vi "sub vi - GET ALL TEMP v7.vi"(0 "LA01-EN":bool, 1 "LA02-EN":bool, 3 "LA03-EN":bool, 4 "LA04-EN":bool, 5 "LA05-EN":bool, 6 "simulate":bool, 7 "Gen Cal Value":dbl) -> (10 "LOOP TIME":dbl, 11 "Fault Counters":u64[](array[numeric]), 12 "ID":T1, 13 "error 1":bool, 14 "LA01 TEMP":T2, 15 "LA02 TEMP":T2, 16 "LA04 TEMP":T2, 17 "LA03 TEMP":T2, 18 "Errors":bool[](array[boolean]), 19 "LA05 TEMP":T2)   [LabVIEW 2017]
uses:
  program files/Global display 4.vi
panel:
  out "error 5":bool
  out "error 4":bool
  out "error 3":bool
  out "error 2":bool
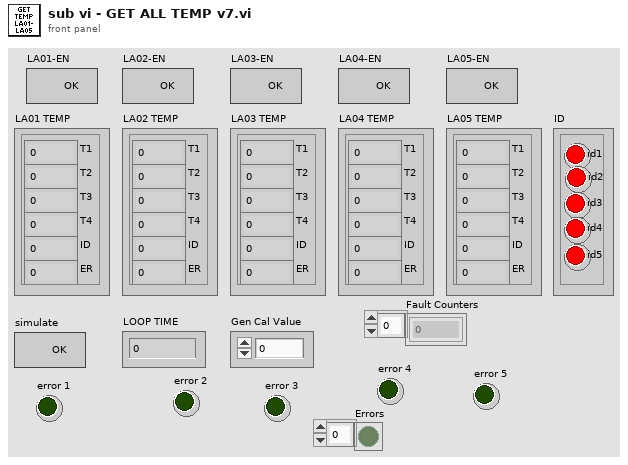
[diagram p1: front panel]
types:
  T1 = cluster{"id1":bool, "id2":bool, "id3":bool, "id4":bool, "id5":bool}
  T2 = cluster{"T1":dbl, "T2":dbl, "T3":dbl, "T4":dbl, "ID":dbl, "ER":dbl}
  T3 = cluster{"1 TL":dbl, "1 TN":dbl, "2 TL":dbl, "2 TN":dbl, "ID":dbl, "ER":dbl}
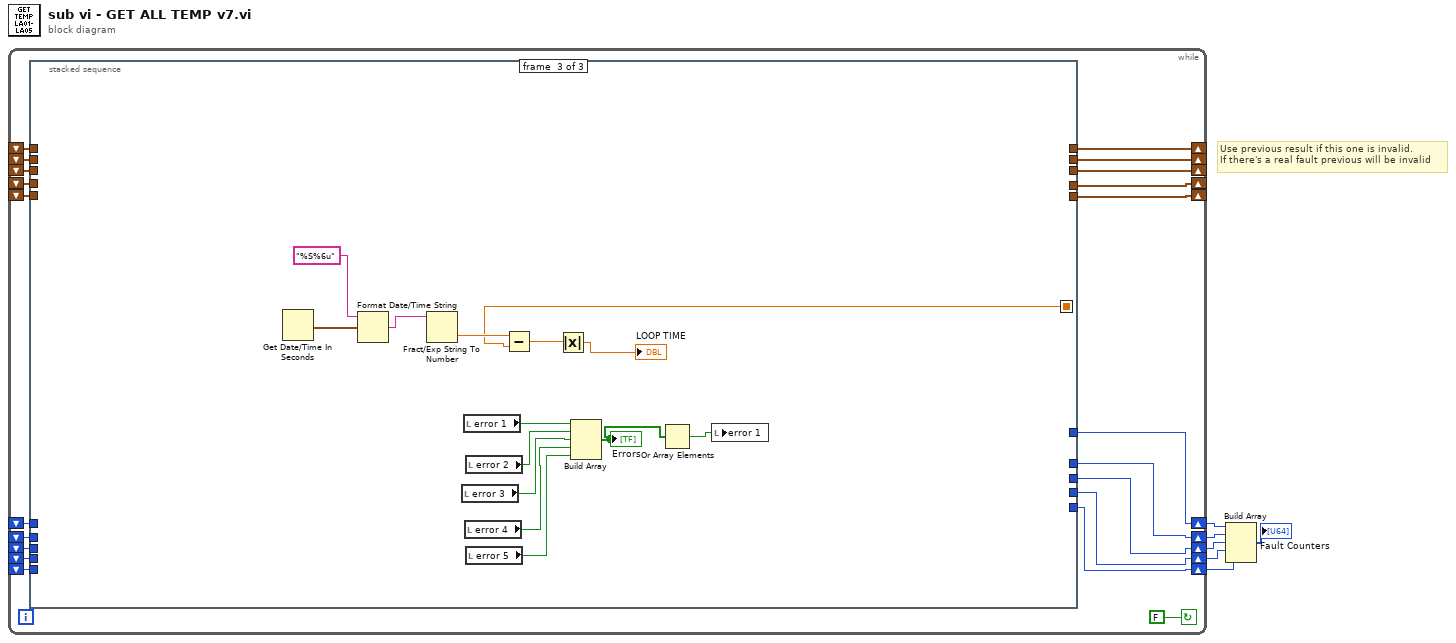
[diagram p0: block diagram]
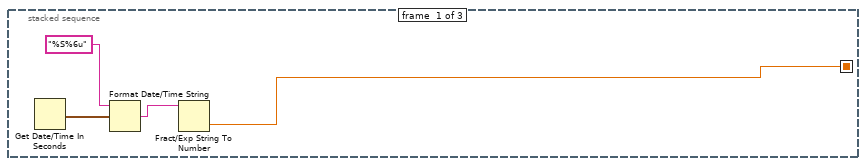
[diagram p2: hidden frame]
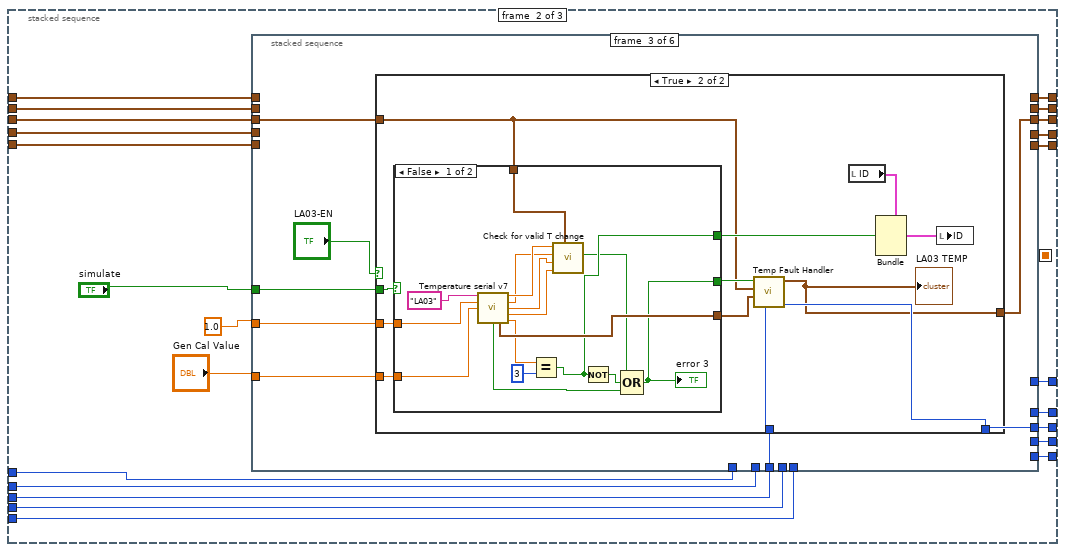
[diagram p3: hidden frame]
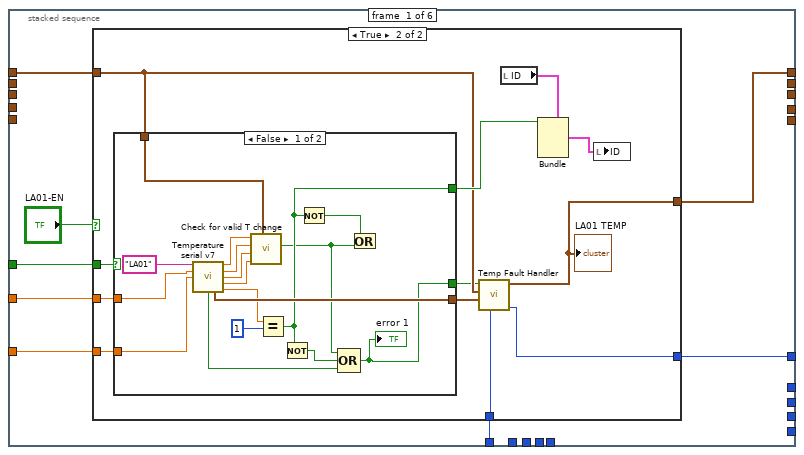
[diagram p4: hidden frame]
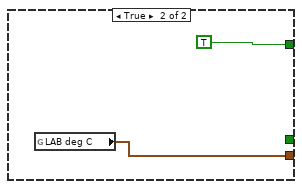
[diagram p6: hidden frame]
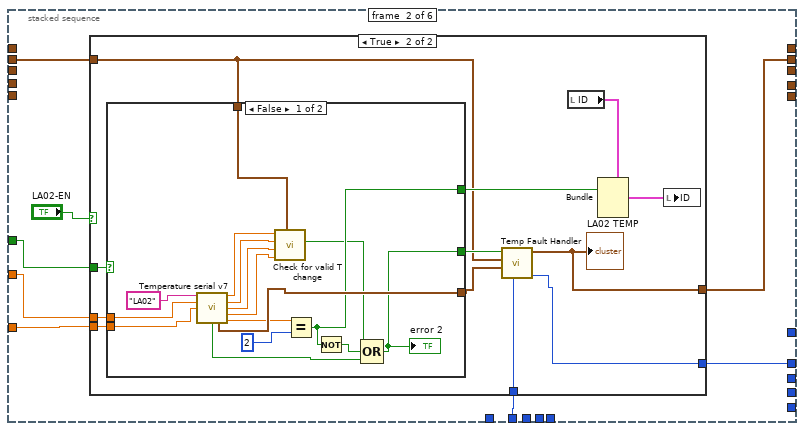
[diagram p7: hidden frame]
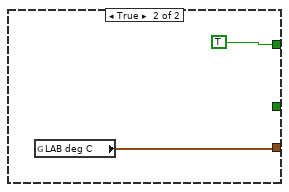
[diagram p9: hidden frame]
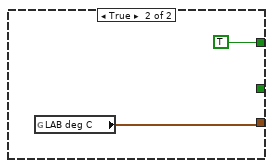
[diagram p11: hidden frame]
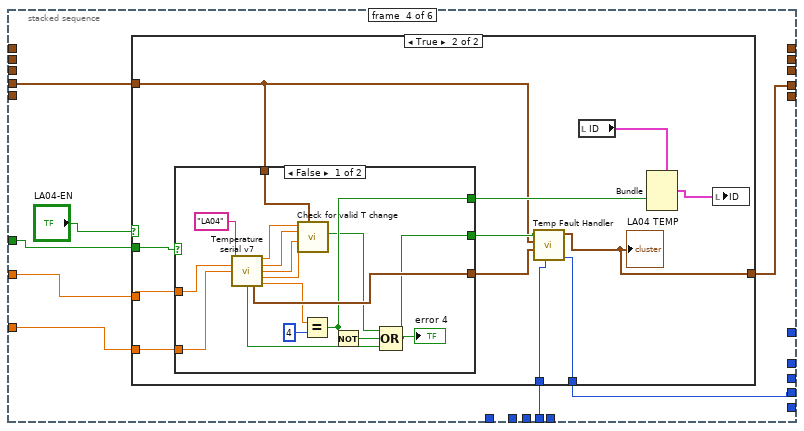
[diagram p12: hidden frame]
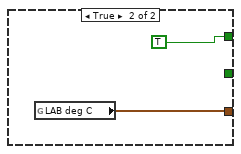
[diagram p14: hidden frame]
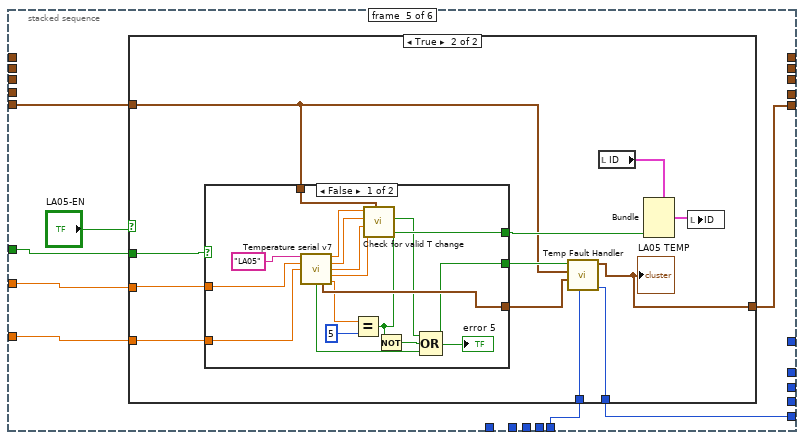
[diagram p15: hidden frame]
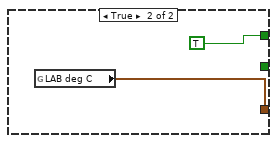
[diagram p17: hidden frame]
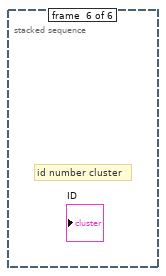
[diagram p18: hidden frame]
diagram:
  # "Use previous result if this one is invalid.\nIf there's a real fault previous will be invalid"
  n1 = while {
    shift-right: [w9] -> w6
    shift-left: _ -> [w26]
    shift-right: [w8] -> w5
    shift-left: _ -> [w25]
    shift-right: [w7] -> w4
    shift-left: _ -> [w24]
    shift-right: [w22] -> _
    shift-left: _ -> [w23]
    shift-right: [w20] -> _
    shift-left: _ -> [w21]
    shift-right: [w18] -> _
    shift-left: _ -> [w19]
    shift-right: [w17] -> _
    shift-left: _ -> [w16]
    shift-right: [w15] -> _
    shift-left: _ -> [w14]
    shift-right: [w11] -> w2
    shift-left: _ -> [w13]
    shift-right: [w10] -> w1
    shift-left: _ -> [w12]
    stop <- FALSE continue-if-true
    n2 = stacked-sequence {
      seq-local: [w28 _ _] -> [_ _ w265]
      tunnel: w26 -> [_ w51 _]
      tunnel: [_ w50 _] -> w9
      tunnel: w25 -> [_ w49 _]
      tunnel: [_ w48 _] -> w8
      tunnel: [_ w47 _] -> w7
      tunnel: w24 -> [_ w46 _]
      tunnel: w23 -> [_ w45 _]
      tunnel: [_ w44 _] -> w22
      tunnel: w21 -> [_ w43 _]
      tunnel: [_ w42 _] -> w20
      tunnel: w19 -> [_ w41 _]
      tunnel: [_ w40 _] -> w18
      tunnel: [_ w39 _] -> w17
      tunnel: w16 -> [_ w38 _]
      tunnel: [_ w37 _] -> w15
      tunnel: w14 -> [_ w36 _]
      tunnel: w13 -> [_ w35 _]
      tunnel: w12 -> [_ w34 _]
      tunnel: [_ w33 _] -> w11
      tunnel: [_ w32 _] -> w10
      frame #0 {
        n3 = Get Date/Time In Seconds() -> (seconds since 1Jan1904=w31:timestamp)
        n4 = Format Date/Time String(time format string (%c)="%S%6u", seconds (now)=w31) -> (date/time string=w29:string)  [unwired: 1 in]
        n5 = Fract/Exp String To Number(string=w29) -> (number=w28:dbl)  [unwired: 3 in, 1 out]
      }
      frame #1 {
        n6 = stacked-sequence {
          tunnel: sgl 1.0 -> [w62 w103 w143 w183 w223 _]
          tunnel: "Gen Cal Value" -> [w61 w102 w142 w182 w222 _]
          tunnel: "simulate" -> [w59 w100 w140 w180 w220 _]
          tunnel: w51 -> [w58 _ _ _ _ _]
          tunnel: [w57 _ _ _ _ _] -> w50
          tunnel: w49 -> [_ w99 _ _ _ _]
          tunnel: [_ w98 _ _ _ _] -> w48
          tunnel: [_ _ w139 _ _ _] -> w47
          tunnel: w46 -> [_ _ w138 _ _ _]
          tunnel: w45 -> [w56 _ _ _ _ _]
          tunnel: [w55 _ _ _ _ _] -> w44
          tunnel: w43 -> [_ w97 _ _ _ _]
          tunnel: [_ w96 _ _ _ _] -> w42
          tunnel: w41 -> [_ _ w137 _ _ _]
          tunnel: [_ _ w136 _ _ _] -> w40
          tunnel: [_ _ _ w179 _ _] -> w39
          tunnel: w38 -> [_ _ _ w178 _ _]
          tunnel: [_ _ _ _ w219 _] -> w37
          tunnel: w36 -> [_ _ _ _ w218 _]
          tunnel: w35 -> [_ _ _ w176 _ _]
          tunnel: w34 -> [_ _ _ _ w217 _]
          tunnel: [_ _ _ w177 _ _] -> w33
          tunnel: [_ _ _ _ w216 _] -> w32
          frame #0 {
            n7 = case shown="True" "LA01-EN" {
              tunnel: w62 -> [_ w76]
              tunnel: w61 -> [_ w75]
              tunnel: w59 -> [_ w74]
              tunnel: w58 -> [w64 w67]
              tunnel: [w64 w66] -> w57
              tunnel: w56 -> [w63 w69]
              tunnel: [w63 w65] -> w55
              frame False {
              }
              frame True {
                n8 = case shown="False" w74 {
                  tunnel: w76 -> [w92 _]
                  tunnel: w75 -> [w91 _]
                  tunnel: [w90 w95] -> w70
                  tunnel: [w80 TRUE] -> w71
                  tunnel: w69 -> [w81 _]
                  tunnel: [w77 _] -> w68
                  frame False {
                    n9 = call "Temperature serial v7.vi"("Command String"="LA01", "Time Out (S)"=w92, "CALIB"=w91) -> ("T1"=w85:dbl, "T2"=w84:dbl, "T3"=w83:dbl, "T4"=w82:dbl, "error"=w88:bool, "output cluster"=w90:cluster{dbl, dbl, dbl, dbl, i32, "error #":dbl}, "Unit ID"=w87:dbl)  [unwired: 6 in]
                    n10 = call "Check for valid T change.vi"("LAB deg C"=w81, "T4"=w82, "T3"=w83, "T2"=w84, "T1"=w85) -> ("Fault"=w78:bool)  [unwired: 6 in]
                    n11 = Equal?(x=w87, y=1) -> (x = y?=w80:bool)
                    n12 = Not(x=w80) -> (.not. x?=w86:bool)
                    n13 = Not(x=w80) -> (.not. x?=w79:bool)
                    n14 = Compound Arithmetic op=OR(w78, w86, w88) -> (w77:bool)
                    "error 1" <- w77
                    n15 = Or(x=w79, y=w78) -> ()  [unwired: 1 out]
                  }
                  frame True {
                    n16 = global read "Global display 4.vi" "LAB deg C"() -> (w95:T3)
                  }
                }
                n17 = call "Temp Fault Handler.vi"("Fault Count In"=w67, "LAB deg C 2"=w70, "LAB deg C Prev"=w69, "Fault"=w68) -> ("Fault Count Out"=w66:u64, "LAB deg C Current"=w65:T3)  [unwired: 6 in]
                "LA01 TEMP" <- w65
                n18 = local read "ID"() -> (w73:T1)
                n19 = Bundle(cluster=w73, "id1"=w71) -> (w72:T1)  [unwired: 4 in]
                n20 = local write "ID"(w72) -> ()
              }
            }
          }
          frame #1 {
            n21 = case shown="True" "LA02-EN" {
              tunnel: w103 -> [_ w117]
              tunnel: w102 -> [_ w116]
              tunnel: w100 -> [_ w115]
              tunnel: w99 -> [w104 w111]
              tunnel: [w104 w107] -> w98
              tunnel: w97 -> [w105 w109]
              tunnel: [w105 w106] -> w96
              frame False {
              }
              frame True {
                n22 = case shown="False" w115 {
                  tunnel: w117 -> [w132 _]
                  tunnel: w116 -> [w131 _]
                  tunnel: [w130 w135] -> w108
                  tunnel: [w125 TRUE] -> w112
                  tunnel: w109 -> [w124 _]
                  tunnel: [w118 _] -> w110
                  frame False {
                    n23 = call "Temperature serial v7.vi"("Command String"="LA02", "Time Out (S)"=w132, "CALIB"=w131) -> ("T1"=w123:dbl, "T2"=w122:dbl, "T3"=w121:dbl, "T4"=w120:dbl, "error"=w129:bool, "output cluster"=w130:cluster{dbl, dbl, dbl, dbl, i32, "error #":dbl}, "Unit ID"=w127:dbl)  [unwired: 6 in]
                    n24 = call "Check for valid T change.vi"("LAB deg C"=w124, "T4"=w120, "T3"=w121, "T2"=w122, "T1"=w123) -> ("Fault"=w119:bool)  [unwired: 6 in]
                    n25 = Equal?(x=w127, y=2) -> (x = y?=w125:bool)
                    n26 = Not(x=w125) -> (.not. x?=w126:bool)
                    n27 = Compound Arithmetic op=OR(w119, w126, w129) -> (w118:bool)
                    "error 2" <- w118
                  }
                  frame True {
                    n28 = global read "Global display 4.vi" "LAB deg C"() -> (w135:T3)
                  }
                }
                n29 = call "Temp Fault Handler.vi"("Fault Count In"=w111, "LAB deg C 2"=w108, "LAB deg C Prev"=w109, "Fault"=w110) -> ("Fault Count Out"=w107:u64, "LAB deg C Current"=w106:T3)  [unwired: 6 in]
                "LA02 TEMP" <- w106
                n30 = local read "ID"() -> (w114:T1)
                n31 = Bundle(cluster=w114, "id2"=w112) -> (w113:T1)  [unwired: 4 in]
                n32 = local write "ID"(w113) -> ()
              }
            }
          }
          frame #2 {
            n33 = case shown="True" "LA03-EN" {
              tunnel: w143 -> [_ w157]
              tunnel: w142 -> [_ w156]
              tunnel: w140 -> [_ w155]
              tunnel: [w145 w147] -> w139
              tunnel: w138 -> [w145 w151]
              tunnel: w137 -> [w144 w149]
              tunnel: [w144 w146] -> w136
              frame False {
              }
              frame True {
                n34 = case shown="False" w155 {
                  tunnel: w157 -> [w172 _]
                  tunnel: w156 -> [w171 _]
                  tunnel: [w170 w175] -> w148
                  tunnel: [w165 TRUE] -> w152
                  tunnel: w149 -> [w164 _]
                  tunnel: [w158 _] -> w150
                  frame False {
                    n35 = call "Temperature serial v7.vi"("Command String"="LA03", "Time Out (S)"=w172, "CALIB"=w171) -> ("T1"=w163:dbl, "T2"=w162:dbl, "T3"=w161:dbl, "T4"=w160:dbl, "error"=w168:bool, "output cluster"=w170:cluster{dbl, dbl, dbl, dbl, i32, "error #":dbl}, "Unit ID"=w167:dbl)  [unwired: 6 in]
                    n36 = Equal?(x=w167, y=3) -> (x = y?=w165:bool)
                    n37 = call "Check for valid T change.vi"("LAB deg C"=w164, "T4"=w160, "T3"=w161, "T2"=w162, "T1"=w163) -> ("Fault"=w159:bool)  [unwired: 6 in]
                    n38 = Not(x=w165) -> (.not. x?=w166:bool)
                    n39 = Compound Arithmetic op=OR(w159, w166, w168) -> (w158:bool)
                    "error 3" <- w158
                  }
                  frame True {
                    n40 = global read "Global display 4.vi" "LAB deg C"() -> (w175:T3)
                  }
                }
                n41 = call "Temp Fault Handler.vi"("Fault Count In"=w151, "LAB deg C 2"=w148, "LAB deg C Prev"=w149, "Fault"=w150) -> ("Fault Count Out"=w147:u64, "LAB deg C Current"=w146:T3)  [unwired: 6 in]
                "LA03 TEMP" <- w146
                n42 = local read "ID"() -> (w154:T1)
                n43 = Bundle(cluster=w154, "id3"=w152) -> (w153:T1)  [unwired: 4 in]
                n44 = local write "ID"(w153) -> ()
              }
            }
          }
          frame #3 {
            n45 = case shown="True" "LA04-EN" {
              tunnel: w183 -> [_ w197]
              tunnel: w182 -> [_ w196]
              tunnel: w180 -> [_ w195]
              tunnel: [w185 w186] -> w179
              tunnel: w178 -> [w185 w190]
              tunnel: [w184 w188] -> w177
              tunnel: w176 -> [w184 w187]
              frame False {
              }
              frame True {
                n46 = case shown="False" w195 {
                  tunnel: w197 -> [w212 _]
                  tunnel: w196 -> [w211 _]
                  tunnel: [w210 w215] -> w189
                  tunnel: [w205 TRUE] -> w192
                  tunnel: w190 -> [w204 _]
                  tunnel: [w198 _] -> w191
                  frame False {
                    n47 = call "Temperature serial v7.vi"("Command String"="LA04", "Time Out (S)"=w212, "CALIB"=w211) -> ("T1"=w203:dbl, "T2"=w202:dbl, "T3"=w201:dbl, "T4"=w200:dbl, "error"=w209:bool, "output cluster"=w210:cluster{dbl, dbl, dbl, dbl, i32, "error #":dbl}, "Unit ID"=w207:dbl)  [unwired: 6 in]
                    n48 = call "Check for valid T change.vi"("LAB deg C"=w204, "T4"=w200, "T3"=w201, "T2"=w202, "T1"=w203) -> ("Fault"=w199:bool)  [unwired: 6 in]
                    n49 = Equal?(x=w207, y=4) -> (x = y?=w205:bool)
                    n50 = Not(x=w205) -> (.not. x?=w206:bool)
                    n51 = Compound Arithmetic op=OR(w199, w206, w209) -> (w198:bool)
                    "error 4" <- w198
                  }
                  frame True {
                    n52 = global read "Global display 4.vi" "LAB deg C"() -> (w215:T3)
                  }
                }
                n53 = call "Temp Fault Handler.vi"("Fault Count In"=w187, "LAB deg C 2"=w189, "LAB deg C Prev"=w190, "Fault"=w191) -> ("Fault Count Out"=w188:u64, "LAB deg C Current"=w186:T3)  [unwired: 6 in]
                "LA04 TEMP" <- w186
                n54 = local read "ID"() -> (w194:T1)
                n55 = Bundle(cluster=w194, "id4"=w192) -> (w193:T1)  [unwired: 4 in]
                n56 = local write "ID"(w193) -> ()
              }
            }
          }
          frame #4 {
            n57 = case shown="True" "LA05-EN" {
              tunnel: w223 -> [_ w237]
              tunnel: w222 -> [_ w236]
              tunnel: w220 -> [_ w235]
              tunnel: [w225 w229] -> w219
              tunnel: w218 -> [w225 w230]
              tunnel: w217 -> [w224 w228]
              tunnel: [w224 w227] -> w216
              frame False {
              }
              frame True {
                n58 = case shown="False" w235 {
                  tunnel: w237 -> [w252 _]
                  tunnel: w236 -> [w251 _]
                  tunnel: [w250 w255] -> w226
                  tunnel: [w245 TRUE] -> w232
                  tunnel: w230 -> [w244 _]
                  tunnel: [w238 _] -> w231
                  frame False {
                    n59 = call "Temperature serial v7.vi"("Command String"="LA05", "Time Out (S)"=w252, "CALIB"=w251) -> ("T1"=w243:dbl, "T2"=w242:dbl, "T3"=w241:dbl, "T4"=w240:dbl, "error"=w249:bool, "output cluster"=w250:cluster{dbl, dbl, dbl, dbl, i32, "error #":dbl}, "Unit ID"=w247:dbl)  [unwired: 6 in]
                    n60 = Equal?(x=w247, y=5) -> (x = y?=w245:bool)
                    n61 = call "Check for valid T change.vi"("LAB deg C"=w244, "T4"=w240, "T3"=w241, "T2"=w242, "T1"=w243) -> ("Fault"=w239:bool)  [unwired: 6 in]
                    n62 = Not(x=w245) -> (.not. x?=w246:bool)
                    n63 = Compound Arithmetic op=OR(w239, w246, w249) -> (w238:bool)
                    "error 5" <- w238
                  }
                  frame True {
                    n64 = global read "Global display 4.vi" "LAB deg C"() -> (w255:T3)
                  }
                }
                n65 = call "Temp Fault Handler.vi"("Fault Count In"=w228, "LAB deg C 2"=w226, "LAB deg C Prev"=w230, "Fault"=w231) -> ("Fault Count Out"=w227:u64, "LAB deg C Current"=w229:T3)  [unwired: 6 in]
                "LA05 TEMP" <- w229
                n66 = local read "ID"() -> (w234:T1)
                n67 = Bundle(cluster=w234, "id5"=w232) -> (w233:T1)  [unwired: 4 in]
                n68 = local write "ID"(w233) -> ()
              }
            }
          }
          frame #5 {
            # "id number cluster"
          }
        }
      }
      frame #2 {
        n69 = Get Date/Time In Seconds() -> (seconds since 1Jan1904=w269:timestamp)
        n70 = Format Date/Time String(time format string (%c)="%S%6u", seconds (now)=w269) -> (date/time string=w267:string)  [unwired: 1 in]
        n71 = Fract/Exp String To Number(string=w267) -> (number=w266:dbl)  [unwired: 3 in, 1 out]
        n72 = local read "error 3"() -> (w260:bool)
        n73 = local read "error 1"() -> (w262:bool)
        n74 = local read "error 4"() -> (w259:bool)
        n75 = local read "error 2"() -> (w261:bool)
        n76 = local read "error 5"() -> (w258:bool)
        n77 = Subtract(x=w266, y=w265) -> (x-y=w264:dbl)
        n78 = Absolute Value(x=w264) -> (abs(x)=→"LOOP TIME":dbl)
        n79 = Build Array(w262, w261, w260, w259, w258) -> (w257:bool[])
        "Errors" <- w257
        n80 = Or Array Elements(Boolean array=w257) -> (logical OR=w256:bool)
        n81 = local write "error 1"(w256) -> ()
      }
    }
  }
  n82 = Build Array(w6, w5, w4, w2, w1) -> (→"Fault Counters":u64[])
